vi "rd_getRecordInfo.vi"(9 "meta in":T1={"TargetFile"=path "", "StreamMode"=enum."File", "Append?"=FALSE, "ChunkSize"=0, "TimeColumnMode"=enum."Empty", "TimestampFormat"="", "AbsoluteTime?"=FALSE, "FileAttribute "={"Creator"="", "Title"="", "SheetName"=""}, "Column"=[], "FileRef"=refnum, "MemoryRef"=[], "RecordInfo"=[], " ChannelPreviousInfo"=[], "ChannelFirstRecord"=[], "PredefinedFormattedValueLength"=20, "DiskTemplate"={"XMLRef"=[refnum, refnum, refnum, refnum, refnum, refnum], "ZipPath"=path "", "MetaFile"={"Ref"=refnum, "NextRow"=0, "NextPosition"=0, "Block"=[]}, "TempFolder"=path ""}}, 10 "start index":u64, 11 "channel index":u32) -> (2 "record index":i32, 3 "record start index":u64)   [LabVIEW 2017, in "NI_ExcelFile.lvlib"]
uses:
  <vilib>/express/express shared/NI_ExcelFile/NI_ExcelFile.lvlib
  <vilib>/express/express shared/NI_ExcelFile/Ctrls/MainData.ctl
  <vilib>/express/express shared/NI_ExcelFile/Ctrls/StreamMode.ctl
  <vilib>/express/express shared/NI_ExcelFile/Ctrls/TimeColumnMode.ctl
  <vilib>/express/express shared/NI_ExcelFile/Ctrls/FileAttribute.ctl
  <vilib>/express/express shared/NI_ExcelFile/Ctrls/Columns.ctl
  <vilib>/express/express shared/NI_ExcelFile/Ctrls/ColumnInfo.ctl
  <vilib>/express/express shared/NI_ExcelFile/Ctrls/DataType.ctl
  <vilib>/express/express shared/NI_ExcelFile/Ctrls/wd_recordInfo.ctl
  <vilib>/express/express shared/NI_ExcelFile/Ctrls/disk_TemplateFile.ctl
  <vilib>/express/express shared/NI_ExcelFile/Ctrls/meta_file.ctl
  <vilib>/express/express shared/NI_ExcelFile/Ctrls/meta_Block.ctl
  <vilib>/express/express shared/NI_ExcelFile/Ctrls/meta_BlockType.ctl
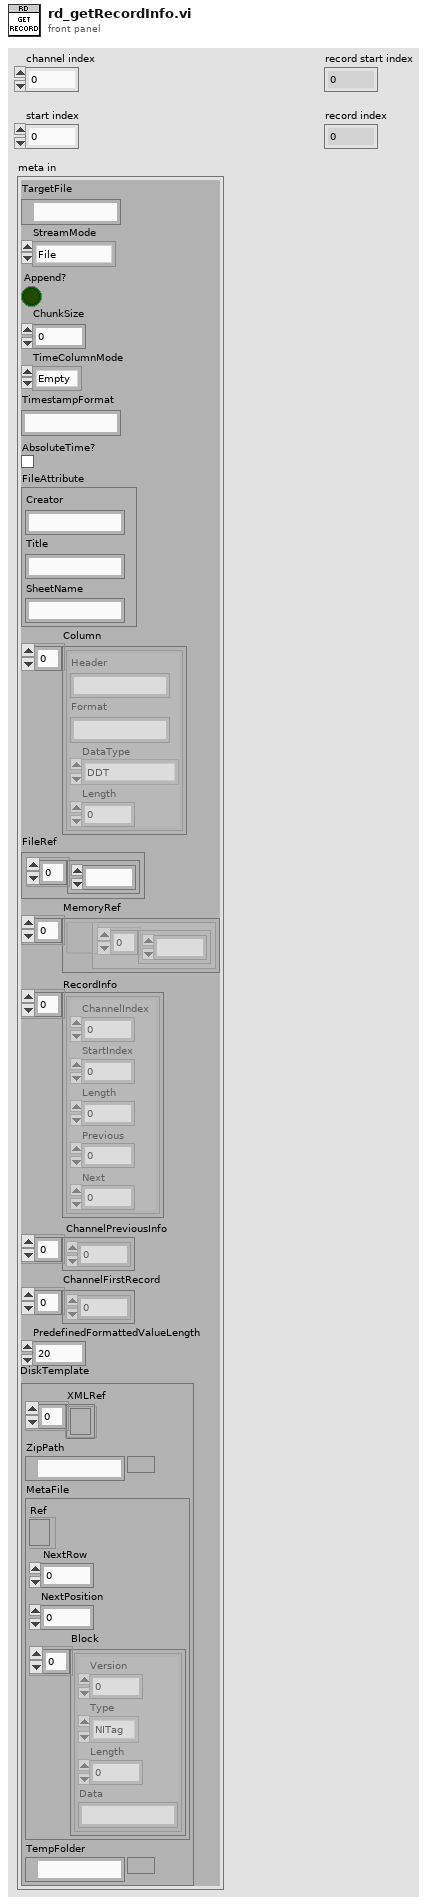
[diagram p1: front panel]
types:
  T1 = typedef "NI_ExcelFile.lvlib/MainData.ctl" = cluster{"TargetFile":path, "StreamMode":T2, "Append?":bool, "ChunkSize":u64, "TimeColumnMode":T3, "TimestampFormat":string, "AbsoluteTime?":bool, "FileAttribute ":T4, "Column":T5, "FileRef":refnum<k1>, "MemoryRef":refnum<data-value>[], "RecordInfo":T8[], " ChannelPreviousInfo":u32[], "ChannelFirstRecord":u32[], "PredefinedFormattedValueLength":i64, "DiskTemplate":T9}
  T2 = typedef "NI_ExcelFile.lvlib/StreamMode.ctl" = enum16{"File", "Memory"}
  T3 = typedef "NI_ExcelFile.lvlib/TimeColumnMode.ctl" = enum16{"Empty", "OnePerCh", "One"}
  T4 = typedef "NI_ExcelFile.lvlib/FileAttribute.ctl" = cluster{"Creator":string, "Title":string, "SheetName":string}
  T5 = typedef "NI_ExcelFile.lvlib/Columns.ctl" = T6[]
  T6 = typedef "NI_ExcelFile.lvlib/ColumnInfo.ctl" = cluster{"Header":string, "Format":string, "DataType":T7, "Length":u64}
  T7 = typedef "NI_ExcelFile.lvlib/DataType.ctl" = enum16{"DDT", "WFM", "Array of STR", "Array of DBL", "Array of I8", "Array of I16", "Array of I32", "Array of I64", "Array of SGL", "Array of U8", "Array of U16", "Array of U32", "Array of U64", "Array of Time"}
  T8 = typedef "NI_ExcelFile.lvlib/wd_recordInfo.ctl" = cluster{"ChannelIndex":u32, "StartIndex":u64, "Length":u64, "Previous":i32, "Next":i32}
  T9 = typedef "NI_ExcelFile.lvlib/disk_TemplateFile.ctl" = cluster{"XMLRef":refnum<file>[], "ZipPath":path, "MetaFile":T10, "TempFolder":path}
  T10 = typedef "NI_ExcelFile.lvlib/meta_file.ctl" = cluster{"Ref":refnum<file>, "NextRow":i32, "NextPosition":i64, "Block":T11[]}
  T11 = typedef "NI_ExcelFile.lvlib/meta_Block.ctl" = cluster{"Version":u16, "Type":T12, "Length":i32, "Data":string}
  T12 = typedef "NI_ExcelFile.lvlib/meta_BlockType.ctl" = enum16{"NITag", "File", "Column"}
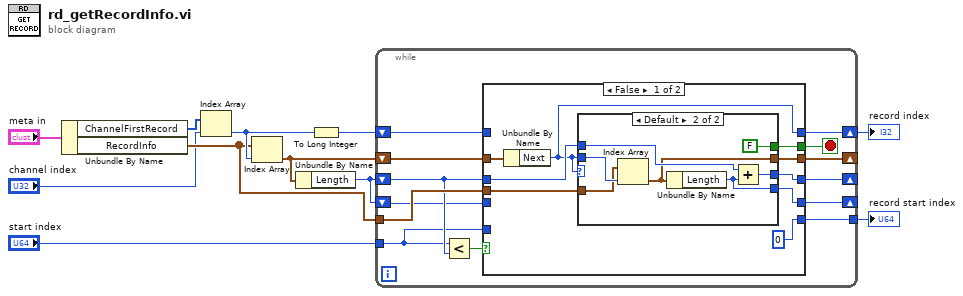
[diagram p0: block diagram]
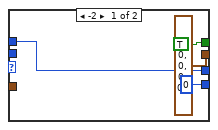
[diagram p2: hidden frame]
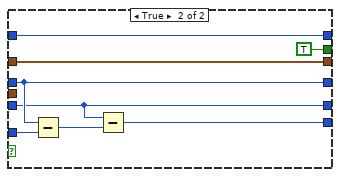
[diagram p3: hidden frame]
diagram:
  n1 = Unbundle By Name("meta in") -> ("ChannelFirstRecord"=w5:u32[], "RecordInfo"=w7:T8[])
  n2 = Index Array(array=w5, index="channel index") -> (element=w10:u32)
  n3 = Index Array(array=w7, index=w10) -> (element=w2:T8)
  n4 = Unbundle By Name(w2) -> ("Length"=w8:u64)
  n5 = To Long Integer(number=w10) -> (32bit integer=w1:i32)
  n6 = while {
    tunnel: "start index" -> [w12]
    shift-right: [w22] -> _
    shift-left: w8 -> [w23]
    tunnel: w7 -> [w24]
    tunnel: [w19] -> w9
    shift-right: [w14] -> _
    shift-left: w2 -> [w16]
    shift-right: [w13] -> _
    shift-left: w8 -> [w20]
    shift-right: [w17] -> w11
    shift-left: w1 -> [w18]
    stop <- w15 stop-if-true
    n7 = Less?(x=w12, y=w23) -> (x < y?=w21:bool)
    n8 = case shown="False" w21 {
      tunnel: w24 -> [w33 _]
      tunnel: w23 -> [w32 w46]
      tunnel: [w31 w46] -> w22
      tunnel: w12 -> [_ w52]
      tunnel: w20 -> [_ w45]
      tunnel: [u64 0 w50] -> w19
      tunnel: w18 -> [_ w49]
      tunnel: [w29 w49] -> w17
      tunnel: w16 -> [w30 w47]
      tunnel: [w28 TRUE] -> w15
      tunnel: [w27 w47] -> w14
      tunnel: [w26 w45] -> w13
      frame False {
        n9 = Unbundle By Name(w30) -> ("Next"=w29:i32)
        n10 = case shown="Default" w29 {
          tunnel: w33 -> [_ w40]
          tunnel: w32 -> [w36 w44]
          tunnel: [w36 w43] -> w31
          tunnel: [T8 {"ChannelIndex"=0, "StartIndex"=0, "Length"=0, "Previous"=0, "Next"=0} ("RecordInfo") w39] -> w27
          tunnel: w29 -> [_ w42]
          tunnel: [TRUE FALSE] -> w28
          tunnel: [u64 0 ("Length") w38] -> w26
          frame -2 {
          }
          frame Default {
            n11 = Index Array(array=w40, index=w42) -> (element=w39:T8)
            n12 = Unbundle By Name(w39) -> ("Length"=w38:u64)
            n13 = Add(x=w44, y=w38) -> (x+y=w43:u64)
          }
        }
      }
      frame True {
        n14 = Subtract(x=w46, y=w52) -> (x-y=w51:u64)
        n15 = Subtract(x=w45, y=w51) -> (x-y=w50:u64)
      }
    }
  }
  "record index" <- w11
  "record start index" <- w9
